vi "ReadMessage.vi"(8 "error in (no error)":errorcluster, 11 "TCP_Client in":refnum<class "TCP_Client.lvclass">) -> (0 "error out":errorcluster, 3 "TCP_Client out":refnum<class "TCP_Client.lvclass">)   [LabVIEW 2023, in "TCP_Client.lvlib" / "TCP_Client.lvclass"]
uses:
  TCP_Client.lvclass
  C:/Program Files (x86)/National Instruments/LabVIEW 2023/vi.lib/ActorFramework/Actor/Actor.lvclass
  <vilib>/ActorFramework/Actor/Actor.lvclass/Actor.ctl
  <vilib>/ActorFramework/Message Enqueuer/Message Enqueuer.lvclass/Message Enqueuer.ctl
  TCP_Client.lvclass/TCP_Client.ctl
  TCP_Client Messages/DisabelConnectButton Msg/DisabelConnectButton Msg.lvclass/DisabelConnectButton Msg.ctl
  <vilib>/ActorFramework/Message Enqueuer/Init from Existing Queue.vi
  <vilib>/ActorFramework/Message Enqueuer/Enqueue.vi
  TCP_Client Messages/LookForStartOfMessage Msg/LookForStartOfMessage Msg.lvclass
  C:/Program Files (x86)/National Instruments/LabVIEW 2023/vi.lib/ActorFramework/Message/Message.lvclass
  TCP_Client Messages/DisabelConnectButton Msg/DisabelConnectButton Msg.lvclass
  <vilib>/ActorFramework/Message Priority Queue/Priority Enqueue.vi
  <vilib>/ActorFramework/Message Enqueuer/Message Enqueuer.lvclass
  <vilib>/ActorFramework/Actor/Actor.lvclass
  TCP_Server_Connection_Handler/TCP_Server_Connection_Handler/TCP_Server_Connection_Handler.lvclass
  TCP_Client Messages/SaveFile Msg/SaveFile Msg.lvclass
  C:/Source/LabVIEW/TCP_server/TCP_Client/TCP_Client/TCP_Client.lvclass
  C:/Source/LabVIEW/TCP_server/SimpleErrorLogger/ApplicationWithErrorLogger/ApplicationWithErrorLogger.lvclass
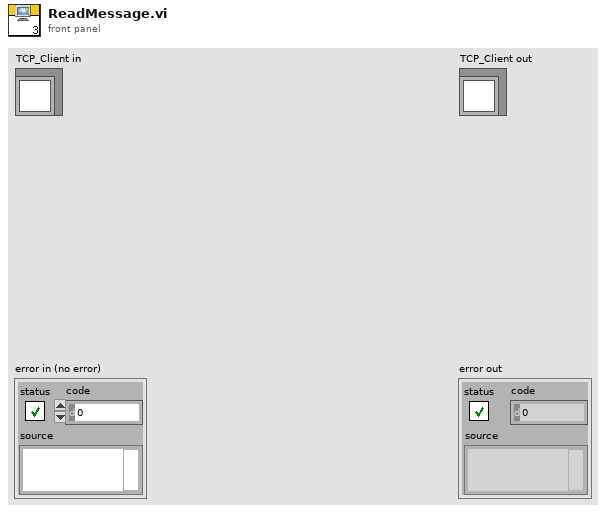
[diagram p1: front panel]
types:
  T1 = enum8{"Enabled", "Disabled", "Disabled and Grayed Out"}
  T2 = typedef "TCP_Server_Connection_Handler.lvlib/messageType.ctl" = enum16{"message", "file", "get"}
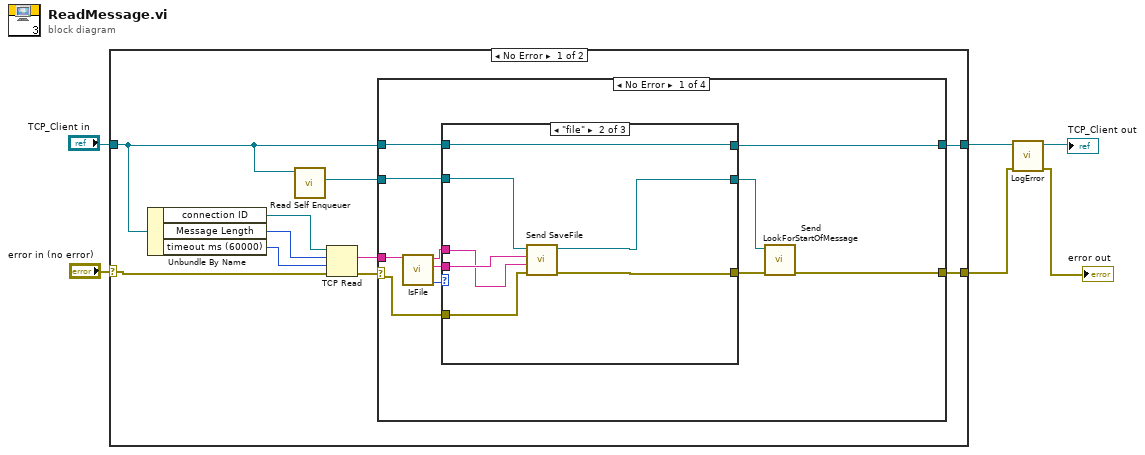
[diagram p0: block diagram]
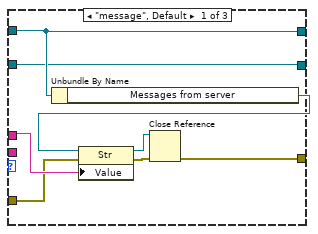
[diagram p2: hidden frame]
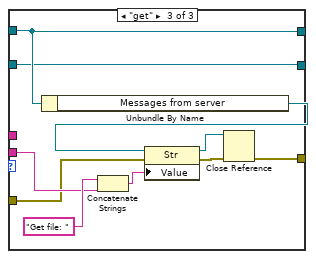
[diagram p3: hidden frame]
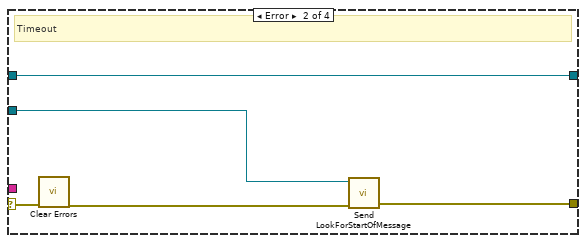
[diagram p4: hidden frame]
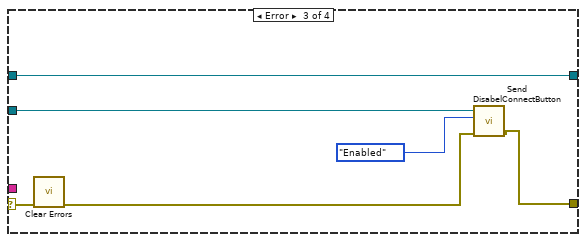
[diagram p5: hidden frame]
diagram:
  n1 = case shown="No Error" "error in (no error)" {
    selector: "error in (no error)" -> [w9 w67]
    tunnel: [w14 w67] -> w2
    tunnel: [w13 w66] -> w4
    tunnel: "TCP_Client in" -> [w8 w66]
    frame No Error {
      n2 = Unbundle By Name(w8) -> ("connection ID"=w12:refnum<k5>, "Message Length"=w10:i32, "timeout ms (60000)"=w11:i32)
      n3 = call <vilib>:"Read Self Enqueuer.vi"("Actor"=w8) -> ("Self Enqueuer"=w7:refnum<class "Message Enqueuer.lvclass">)  [unwired: 10 in]
      n4 = TCP Read(connection ID=w12, bytes to read=w10, error in (no error)=w9, 9:w11) -> (data out=w15:string, error out=w16:errorcluster)  [unwired: 1 in, 1 out]
      n5 = case shown="No Error" w16 {
        selector: w16 -> [w20 w56 w62 w65]
        tunnel: w15 -> [w25 _ _ _]
        tunnel: w8 -> [w27 w53 w58 w64]
        tunnel: [w17 w54 w60 w65] -> w14
        tunnel: [w21 w53 w58 w64] -> w13
        tunnel: w7 -> [w26 w57 w63 _]
        frame No Error {
          n6 = call "IsFile.vi"("message in"=w25) -> ("Message type out"=w24:T2, "Filename"=w22:string, "message/data out"=w23:string)  [unwired: 8 in]
          n7 = case shown="\"file\"" w24 {
            tunnel: [w32 w37 w44] -> w18
            tunnel: w27 -> [w30 w42 w52]
            tunnel: w26 -> [w28 w41 w43]
            tunnel: w23 -> [w31 w38 _]
            tunnel: w22 -> [_ w39 w49]
            tunnel: [w30 w42 w52] -> w21
            tunnel: w20 -> [w29 w40 w45]
            tunnel: [w28 w36 w43] -> w19
            frame "message", Default {
              n8 = Unbundle By Name(w30) -> ("Messages from server"=w35:refnum<vi>)
              n9 = property class="Str"(reference=w35, error in=w29, "Value"=w31) -> (reference out=w33:refnum<vi>, error out=w34:errorcluster)
              n10 = Close Reference(reference=w33, error in (no error)=w34) -> (error out=w32:errorcluster)
            }
            frame "file" {
              n11 = call "Send SaveFile.vi"("error in (no error)"=w40, "Data"=w38, "Filename"=w39, "Message Enqueuer"=w41) -> ("error out"=w37:errorcluster, "Message Enqueuer out"=w36:refnum<class "Message Enqueuer.lvclass">)  [unwired: 6 in]
            }
            frame "get" {
              n12 = Unbundle By Name(w52) -> ("Messages from server"=w51:refnum<vi>)
              n13 = Concatenate Strings("Get file: ", w49) -> (w48:string)
              n14 = property class="Str"(reference=w51, error in=w45, "Value"=w48) -> (reference out=w46:refnum<vi>, error out=w47:errorcluster)
              n15 = Close Reference(reference=w46, error in (no error)=w47) -> (error out=w44:errorcluster)
            }
          }
          n16 = call "Send LookForStartOfMessage.vi"("error in (no error)"=w18, "Message Enqueuer"=w19) -> ("error out"=w17:errorcluster)  [unwired: 8 in, 1 out]
        }
        frame Error {
          # "Timeout"
          n17 = call <vilib>:"Clear Errors.vi"("error in (no error)"=w56) -> ("error out"=w55:errorcluster)  [unwired: 5 in, 1 out]
          n18 = call "Send LookForStartOfMessage.vi"("error in (no error)"=w55, "Message Enqueuer"=w57) -> ("error out"=w54:errorcluster)  [unwired: 8 in, 1 out]
        }
        frame Error {
          n19 = call <vilib>:"Clear Errors.vi"("error in (no error)"=w62) -> ("error out"=w61:errorcluster)  [unwired: 5 in, 1 out]
          n20 = call "Send DisabelConnectButton.vi"("error in (no error)"=w61, "Connect button Disabled"=T1."Enabled", "Message Enqueuer"=w63) -> ("error out"=w60:errorcluster)  [unwired: 7 in, 1 out]
        }
        frame Default {
        }
      }
    }
    frame Error {
    }
  }
  n21 = call "LogError.vi"("error in (no error)"=w2, "TCP_Client in"=w4) -> ("error out"=→"error out":errorcluster, "TCP_Client out"=→"TCP_Client out":refnum<class "TCP_Client.lvclass">)  [unwired: 8 in]
